vi "setTriggerMode.vi"(8 "error in (no error)":errorcluster, 9 "Path":path, 10 "triggerMode":i32, 11 "CameraManager in":refnum<class "CameraManager.lvclass">) -> (0 "error out":errorcluster, 3 "CameraManager out":refnum<class "CameraManager.lvclass">)   [LabVIEW 2011, in "iManagement.lvlib" / "CameraManager.lvclass"]
uses:
  CameraManager.lvclass
  CameraManager.lvclass/CameraManager.ctl
  Hal/Channels/Camera/CameraController.lvclass
  Hal/Channels/Camera/CameraEventsManager/CameraEventsManger.lvclass
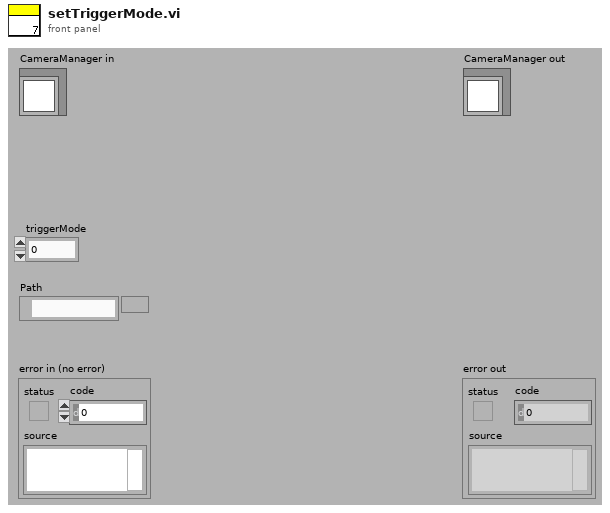
[diagram p1: front panel]
types:
  T1 = cluster{"settingsFrontEndEvents":cluster{"loadSettingsFromPath":refnum<user-event>, "lookUpElementEvent":refnum<user-event>, "saveSettings":refnum<user-event>, "loadSettings":refnum<user-event>, "close":refnum<user-event>, "replaceElement":refnum<user-event>, "findParentNodes":refnum<user-event>, "createNode":refnum<user-event>}, "settingBackEndEvents":cluster{"defaultSettingsPathRequest":refnum<user-event>, "searchResultEvent":refnum<user-event>, "settingsSaved":refnum<user-event>, "settingsLoaded":refnum<user-event>, "foundParentNode":refnum<user-event>}}
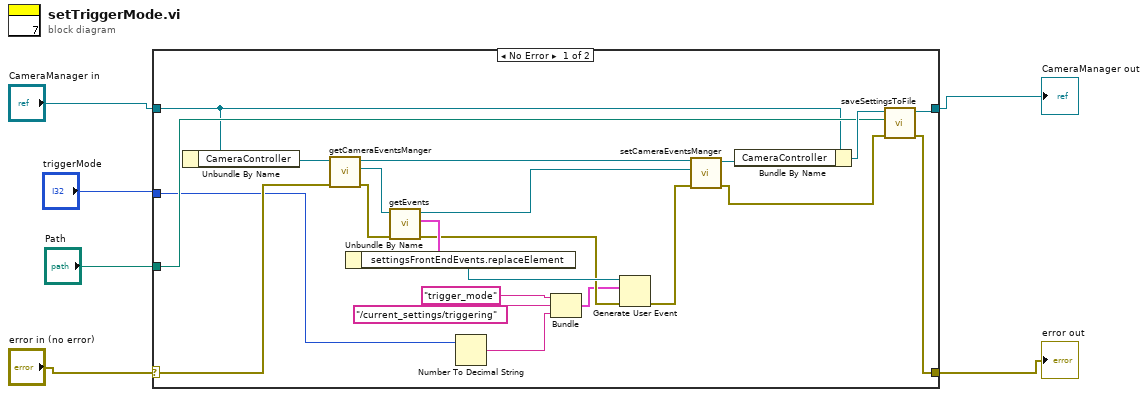
[diagram p0: block diagram]
diagram:
  n1 = case shown="No Error" "error in (no error)" {
    selector: "error in (no error)" -> [w23 w30]
    tunnel: [w13 w30] -> w4
    tunnel: [w16 w29] -> w5
    tunnel: "CameraManager in" -> [w12 w29]
    tunnel: "triggerMode" -> [w9 _]
    tunnel: "Path" -> [w15 _]
    frame No Error {
      n2 = Unbundle By Name(w12) -> ("CameraController"=w26:refnum<class "CameraController.lvclass">)
      n3 = call-dynamic "getCameraEventsManger.vi"("error in (no error)"=w23, "CameraController.lvclass in"=w26) -> ("error out"=w27:errorcluster, "Hardware:Channels.lvlib:CameraEventsManger.lvclass"=w28:refnum<class "CameraEventsManger.lvclass">, "CameraController.lvclass out"=w25:refnum<class "CameraController.lvclass">)  [unwired: 7 in]
      n4 = call-dynamic "getEvents.vi"("error in (no error)"=w27, "CameraEventsManger in"=w28) -> ("error out"=w19:errorcluster, "settingsEvents"=w21:T1, "CameraEventsManger out"=w22:refnum<class "CameraEventsManger.lvclass">)  [unwired: 5 in, 2 out]
      n5 = Unbundle By Name(w21) -> ("settingsFrontEndEvents.replaceElement"=w20:refnum<user-event>)
      n6 = Number To Decimal String(number=w9) -> (decimal integer string=w8:string)  [unwired: 1 in]
      n7 = Bundle("trigger_mode", "/current_settings/triggering", w8) -> (w7:cluster{string, string, string})  [unwired: 1 in]
      n8 = Generate User Event(user event=w20, event data cluster=w7, error in=w19) -> (error out=w18:errorcluster)  [unwired: 1 out]
      n9 = call-dynamic "setCameraEventsManger.vi"("error in (no error)"=w18, "Hardware:Channels.lvlib:CameraEventsManger.lvclass"=w22, "CameraController.lvclass in"=w25) -> ("error out"=w14:errorcluster, "CameraController.lvclass out"=w24:refnum<class "CameraController.lvclass">)  [unwired: 7 in]
      n10 = Bundle By Name(cluster=w12, "CameraController"=w24) -> (w17:refnum<class "CameraManager.lvclass">)
      n11 = call "saveSettingsToFile.vi"("error in (no error)"=w14, "Path"=w15, "CameraManager in"=w17) -> ("error out"=w13:errorcluster, "CameraManager out"=w16:refnum<class "CameraManager.lvclass">)  [unwired: 7 in]
    }
    frame Error {
    }
  }
  "error out" <- w4
  "CameraManager out" <- w5
